vi "TA_Read_Data_3.vi"(11 "File Path":path=path "\\\\Mac\\Home/Desktop/fs-TA/Data/demo_fsta.dat") -> (3 "TA Data":T1)   [LabVIEW 2025]
uses:
  <vilib>/Utility/file.llb/Read Delimited Spreadsheet (DBL).vi
panel:
  out "size (raw data)":i32[](array[numeric])
  out "raw data":dbl[][](array[numeric]) format="%#_8g"
  in  "delimiter (\\t tab; , comma)":string="\t"
  in  "transpose? (F)":bool
  in  "max characters/row  (no limit:0)":i32
  in  "start of read offset (chars.:0)":i32
  in  "number of rows (all:-1)":i32=-1
  in  "format (%.8f)":string="%.8f"
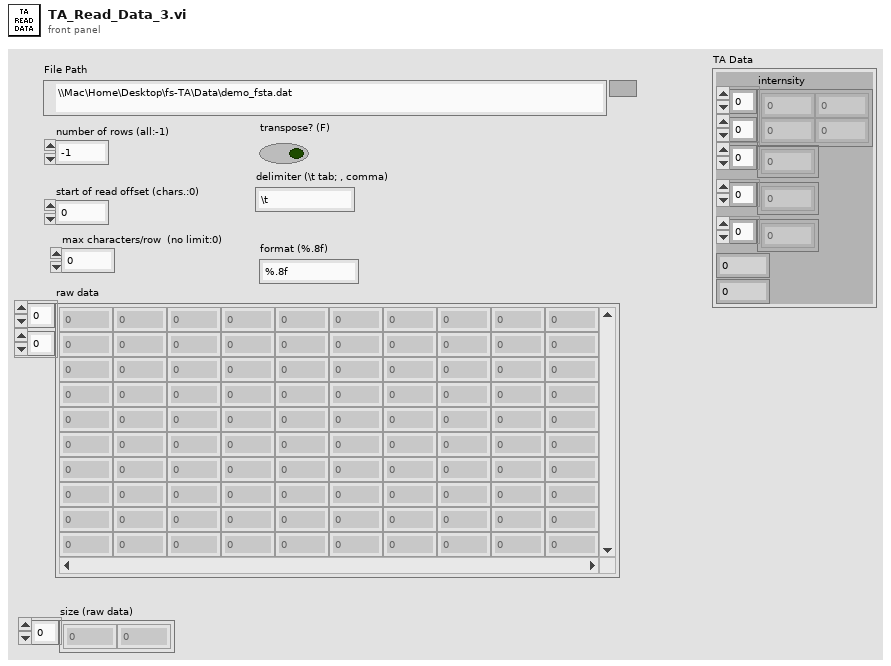
[diagram p1: front panel]
types:
  T1 = cluster{"internsity":dbl[][], dbl[], dbl[], i32[], i32, i32}
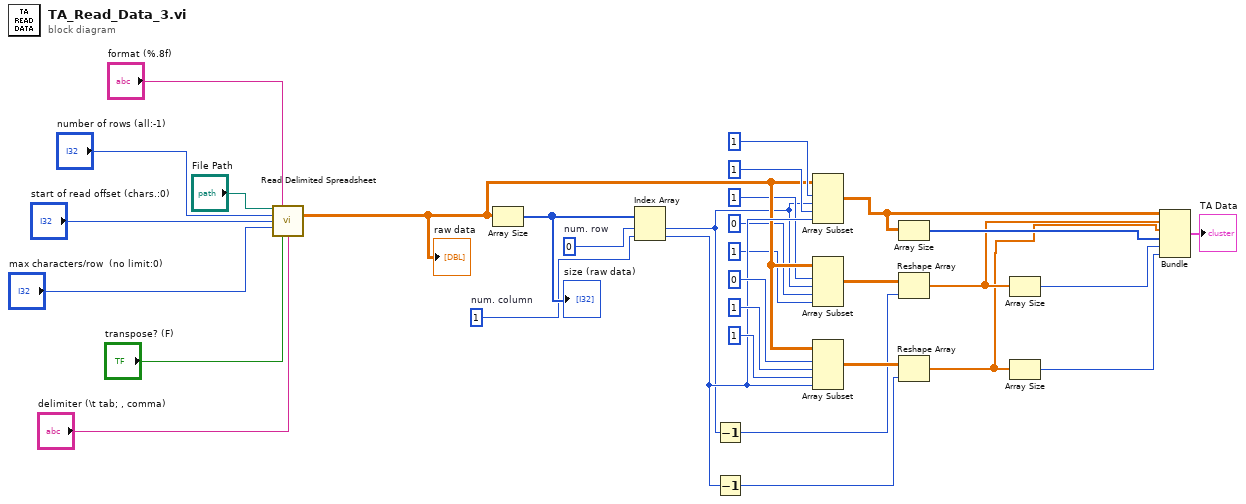
[diagram p0: block diagram]
diagram:
  w18 = 1  # num. column
  w25 = 0  # num. row
  n1 = call-poly <vilib>:"Read Delimited Spreadsheet.vi"("file path (dialog if empty)"="File Path", "format (%.3f)"="format (%.8f)", "number of rows (all:-1)"="number of rows (all:-1)", "start of read offset (chars.:0)"="start of read offset (chars.:0)", "max characters/row  (no limit:0)"="max characters/row  (no limit:0)", "transpose? (F)"="transpose? (F)", "delimiter (\\t)"="delimiter (\\t tab; , comma)") -> ("all rows"=w12:dbl[][])  [unwired: 3 in, 5 out]
  "raw data" <- w12
  n2 = Array Size(array=w12) -> (size(s)=w22:i32[])
  "size (raw data)" <- w22
  n3 = Index Array "Index Array"(array=w22, index #1=w25, index #2=w18) -> (element #1=w8:i32, element #2=w16:i32)
  n4 = Decrement(x=w8) -> (x-1=w14:i32)
  n5 = Decrement(x=w16) -> (x-1=w15:i32)
  n6 = Array Subset "Array Subset"(array=w12, index (row)=1 ("index"), length (row)=w8, index (col)=1 ("index"), length (col)=w16) -> (w4:dbl[][])
  n7 = Array Subset "Array Subset"(array=w12, index (row)=1 ("index"), length (row)=w8, index (col)=0 ("index"), length (col)=1 ("length")) -> (w13:dbl[][])
  n8 = Array Subset "Array Subset"(array=w12, index (row)=0 ("index"), length (row)=1 ("length"), index (col)=1 ("index"), length (col)=w16) -> (w21:dbl[][])
  n9 = Array Size(array=w4) -> (size(s)=w7:i32[])
  n10 = Reshape Array "Reshape Array"(w13, w14) -> (w3:dbl[])
  n11 = Reshape Array "Reshape Array"(w21, w15) -> (w2:dbl[])
  n12 = Array Size(array=w3) -> (size(s)=w6:i32)
  n13 = Array Size(array=w2) -> (size(s)=w5:i32)
  n14 = Bundle(w4, w3, w2, w7, w6, w5) -> (→"TA Data":cluster{dbl[][], dbl[], dbl[], i32[], i32, i32})  [unwired: 1 in]
